vi "FW Arduino Rd Wr Settings.vi"(8 "error in (no error)":errorcluster, 10 "Write? (F:Read)":bool, 11 "Settings":refnum<class "FW Arduino Control.lvclass">) -> (0 "error out":errorcluster, 3 "Settings":refnum<class "FW Arduino Control.lvclass">)   [LabVIEW 2021, in "FW Arduino Control.lvclass"]
uses:
  FW Arduino Control.lvclass
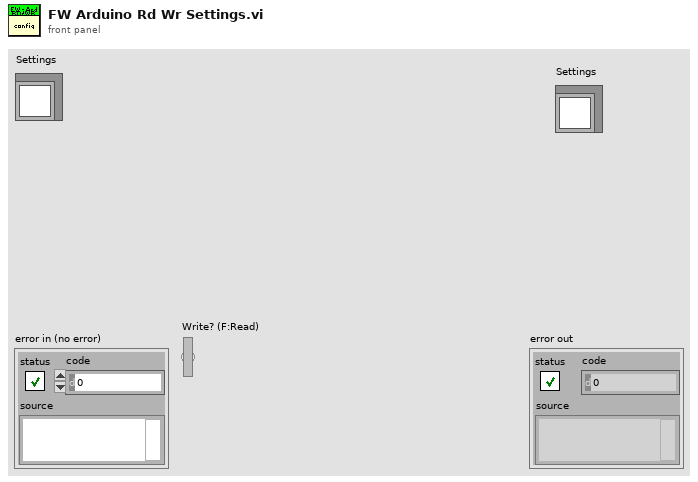
[diagram p1: front panel]
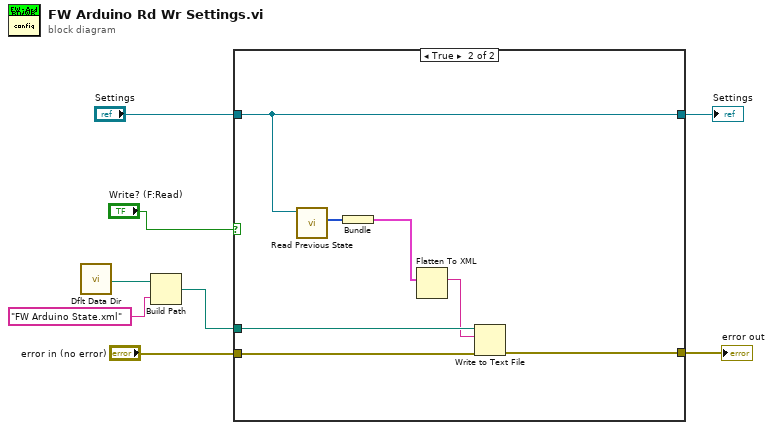
[diagram p0: block diagram]
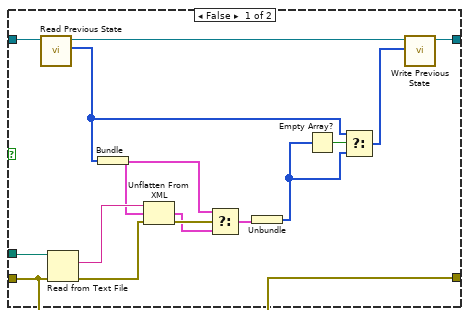
[diagram p2: hidden frame]
diagram:
  n1 = call <vilib>:"Dflt Data Dir.vi"() -> ("App:Default Data Directory"=w5:path)
  n2 = Build Path(base path=w5, name or relative path="FW Arduino State.xml") -> (appended path=w4:path)
  n3 = case shown="True" "Write? (F:Read)" {
    tunnel: "error in (no error)" -> [w19 w30]
    tunnel: "Settings" -> [w18 w26]
    tunnel: w4 -> [w23 w29]
    tunnel: [w19 w27] -> w3
    tunnel: [w13 w26] -> w2
    frame False {
      n4 = call-dynamic "Read Previous State.vi"("FW Arduino Control in"=w18) -> ("Previous State"=w11:i32[], "FW Arduino Control out"=w14:refnum<class "FW Arduino Control.lvclass">)  [unwired: 8 in, 1 out]
      n5 = Read from Text File(file (use dialog)=w23, error in=w19) -> (text=w22:string, error out=w21:errorcluster)  [unwired: 2 in, 2 out]
      n6 = Bundle("Previous State"=w11) -> (w17:cluster{"Previous State":i32[]})  [unwired: 1 in]
      n7 = Unflatten From XML(xml string=w22, type=w17, error in (no error)=w21) -> (value=w16:cluster{"Previous State":i32[]}, error out=w20:errorcluster)
      n8 = Select(t=w17, s=w20, f=w16) -> (s? t:f=w15:cluster{"Previous State":i32[]})
      n9 = Unbundle(w15) -> ("Previous State"=w10:i32[])
      n10 = Empty Array?(array=w10) -> (empty?=w12:bool)
      n11 = Select(t=w11, s=w12, f=w10) -> (s? t:f=w9:i32[])
      n12 = call-dynamic "Write Previous State.vi"("Previous State"=w9, "FW Arduino Control in"=w14) -> ("FW Arduino Control out"=w13:refnum<class "FW Arduino Control.lvclass">)  [unwired: 8 in, 1 out]
    }
    frame True {
      n13 = call-dynamic "Read Previous State.vi"("FW Arduino Control in"=w26) -> ("Previous State"=w25:i32[])  [unwired: 8 in, 2 out]
      n14 = Bundle("Previous State"=w25) -> (w24:cluster{"Previous State":i32[]})  [unwired: 1 in]
      n15 = Flatten To XML(6:w24) -> (2:w28:string)
      n16 = Write to Text File(file (use dialog)=w29, text=w28, error in=w30) -> (error out=w27:errorcluster)  [unwired: 1 in, 2 out]
    }
  }
  "error out" <- w3
  "Settings" <- w2
